vi "Helper - ExitLine to Wpts.vi"(6 "NorthOut":dbl, 7 "Next Point":T1 {"East" format="%#_5g"}, 9 "East Out":dbl, 10 "Best Angle":dbl, 11 "Distance":dbl) -> (3 "Point on Line":dbl[][](array[numeric]))   [LabVIEW 2011]
doc: "This VI creates 5 points on two differents lines. Those lines are in a certain angle (45/-45 deg off the line Startpoint-Endpoint), starting at the endpoint. \nThe 5 points on each line divide the line with a length that is equal to the distance SP - EP into five qual parts. \nAfter the points are created, the VI compares both lines and selects the one that is further away from the next waypoint. This ensures, that the point is created on the right side for the desired buoy rounding direction.\nThe output is a 2D array with five rows for each point and two colums for X and Y position of the points."
uses:
  2 Typedefs/Velocity.ctl
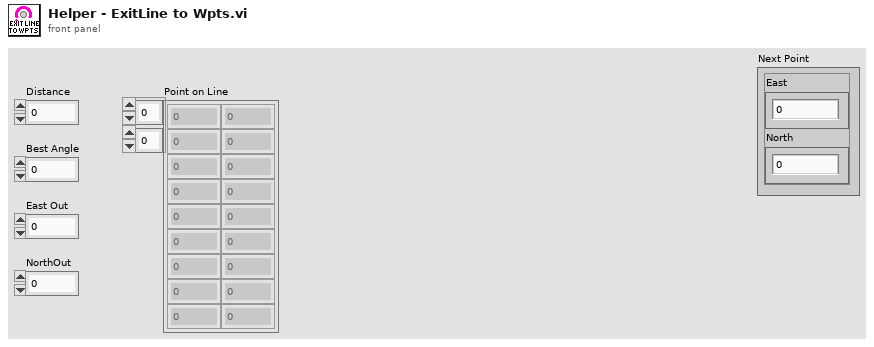
[diagram p1: front panel]
types:
  T1 = typedef "Velocity.ctl" = cluster{"East":dbl, "North":dbl}
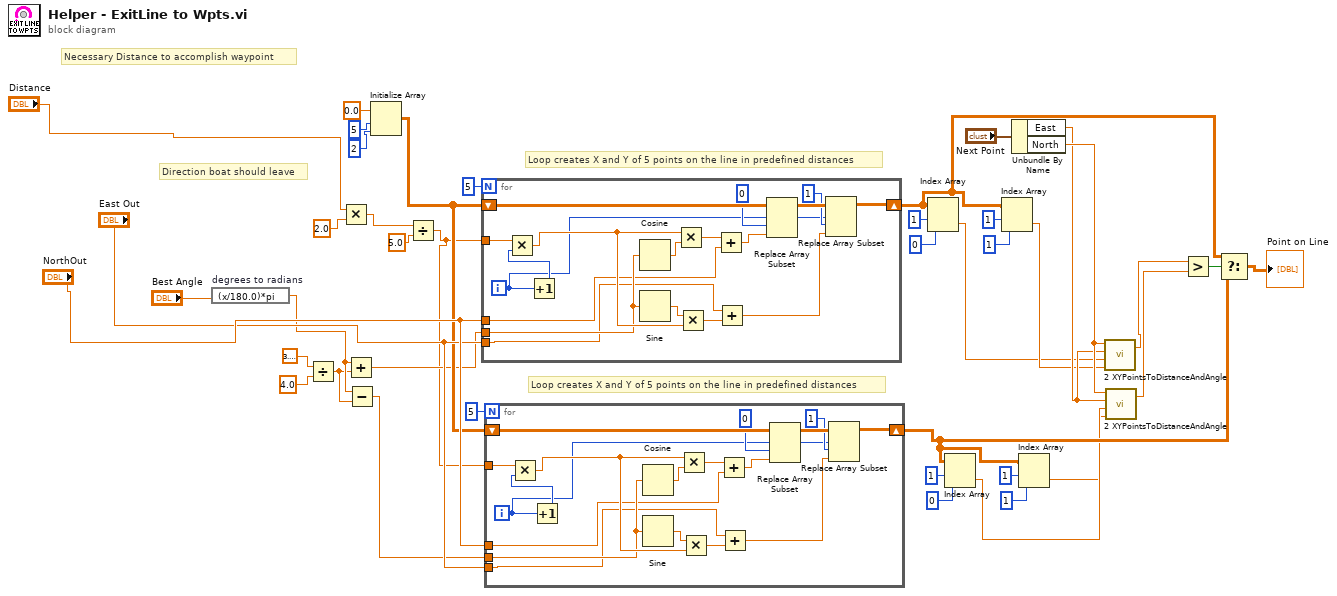
[diagram p0: block diagram]
diagram:
  # "Loop creates X and Y of 5 points on the line in predefined distances"
  # "Loop creates X and Y of 5 points on the line in predefined distances"
  # "Direction boat should leave"
  # "Necessary Distance to accomplish waypoint"
  n1 = expression code="(x/180.0)*pi" "degrees to radians"("Best Angle") -> (w27:dbl)
  n2 = Divide(x=3.141592653589793, y=4.0) -> (x/y=w26:dbl)
  n3 = Multiply(x="Distance", y=2.0) -> (x*y=w35:dbl)
  n4 = Add(x=w27, y=w26) -> (x+y=w16:dbl)
  n5 = Subtract(x=w27, y=w26) -> (x-y=w15:dbl)
  n6 = Initialize Array(0.0, 5, 2) -> (w17:dbl[][])
  n7 = Divide(x=w35, y=5.0) -> (x/y=w11:dbl)
  n8 = for {
    N: 5 -> [_]
    tunnel: w11 -> [w58]
    shift-right: [w47] -> w14
    shift-left: w17 -> [w57]
    tunnel: w16 -> [w53]
    tunnel: "NorthOut" -> [w50]
    tunnel: "East Out" -> [w49]
    i -> [w44]
    n9 = Increment(x=w44) -> (x+1=w59:i32)
    n10 = Multiply(x=w58, y=w59) -> (x*y=w54:dbl)
    n11 = Cosine(x=w53) -> (cos(x)=w56:dbl)
    n12 = Sine(x=w53) -> (sin(x)=w55:dbl)
    n13 = Multiply(x=w54, y=w56) -> (x*y=w52:dbl)
    n14 = Multiply(x=w55, y=w54) -> (x*y=w51:dbl)
    n15 = Add(x=w52, y=w50) -> (x+y=w43:dbl)
    n16 = Add(x=w49, y=w51) -> (x+y=w42:dbl)
    n17 = Replace Array Subset(array=w57, new element=w43, index (row)=w44, index (col)=0) -> (w48:dbl[][])
    n18 = Replace Array Subset(array=w48, new element=w42, index (row)=w44, index (col)=1) -> (w47:dbl[][])
  }
  n19 = for {
    N: 5 -> [_]
    tunnel: w11 -> [w76]
    shift-right: [w65] -> w13
    shift-left: w17 -> [w75]
    tunnel: w15 -> [w71]
    tunnel: "NorthOut" -> [w68]
    tunnel: "East Out" -> [w67]
    i -> [w62]
    n20 = Increment(x=w62) -> (x+1=w77:i32)
    n21 = Multiply(x=w76, y=w77) -> (x*y=w72:dbl)
    n22 = Cosine(x=w71) -> (cos(x)=w74:dbl)
    n23 = Sine(x=w71) -> (sin(x)=w73:dbl)
    n24 = Multiply(x=w72, y=w74) -> (x*y=w70:dbl)
    n25 = Multiply(x=w73, y=w72) -> (x*y=w69:dbl)
    n26 = Add(x=w70, y=w68) -> (x+y=w61:dbl)
    n27 = Add(x=w67, y=w69) -> (x+y=w60:dbl)
    n28 = Replace Array Subset(array=w75, new element=w61, index (row)=w62, index (col)=0) -> (w66:dbl[][])
    n29 = Replace Array Subset(array=w66, new element=w60, index (row)=w62, index (col)=1) -> (w65:dbl[][])
  }
  n30 = Index Array(array=w14, index (row)=1, index (col)=0) -> (element=w6:dbl)
  n31 = Index Array(array=w13, index (row)=1, index (col)=0) -> (element=w5:dbl)
  n32 = Index Array(array=w14, index (row)=1, index (col)=1) -> (element=w7:dbl)
  n33 = Unbundle By Name("Next Point") -> ("East"=w8:dbl, "North"=w9:dbl)
  n34 = Index Array(array=w13, index (row)=1, index (col)=1) -> (element=w4:dbl)
  n35 = call "2 XYPointsToDistanceAndAngle.vi"("East 2"=w7, "North 2"=w6, "East 1"=w8, "North 1"=w9) -> ("Distance"=w2:dbl)  [unwired: 1 out]
  n36 = call "2 XYPointsToDistanceAndAngle.vi"("East 2"=w4, "North 2"=w5, "East 1"=w8, "North 1"=w9) -> ("Distance"=w3:dbl)  [unwired: 1 out]
  n37 = Greater?(x=w2, y=w3) -> (0:w1:bool)
  n38 = Select(t=w14, s=w1, f=w13) -> (s? t:f=→"Point on Line":dbl[][])
